vi "8_Find roots of the quadratic equation.vi"() -> ()   [LabVIEW 2018]
panel:
  out "SUBTRACT":dbl
  out "ADD":dbl
  in  "C":dbl
  in  "B":dbl
  in  "A":dbl
  # "WAP to find roots of the quadratic equation"
  # "Ax^2 + Bx + C= 0"
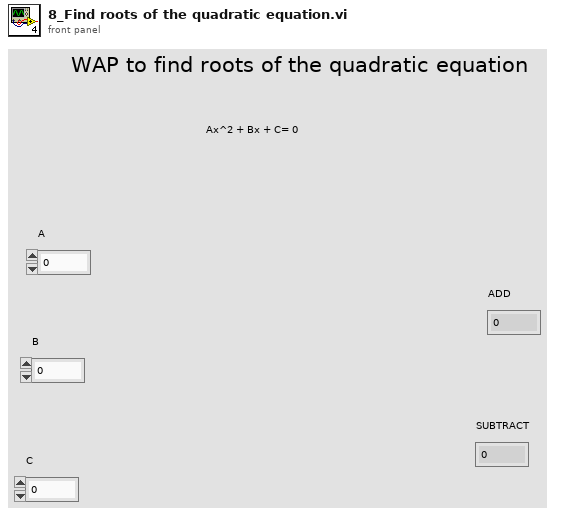
[diagram p1: front panel]
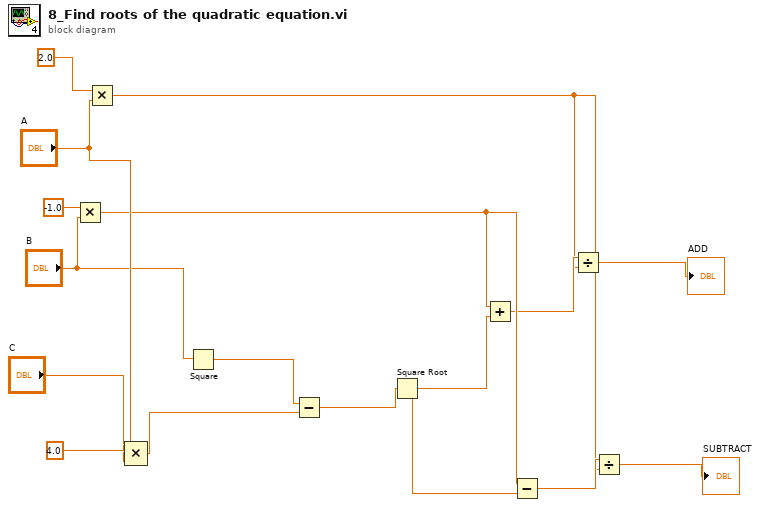
[diagram p0: block diagram]
diagram:
  n1 = Multiply(x=-1.0, y="B") -> (x*y=w6:dbl)
  n2 = Multiply(x=2.0, y="A") -> (x*y=w3:dbl)
  n3 = Compound Arithmetic op=MULTIPLY(4.0 ("result"), "A", "C") -> (w13:dbl)
  n4 = Square(x="B") -> (x^2=w14:dbl)
  n5 = Subtract(x=w14, y=w13) -> (x-y=w12:dbl)
  n6 = Square Root(x=w12) -> (sqrt(x)=w11:dbl)
  n7 = Add(x=w6, y=w11) -> (x+y=w5:dbl)
  n8 = Subtract(x=w6, y=w11) -> (x-y=w4:dbl)
  n9 = Divide(x=w5, y=w3) -> (x/y=→"ADD":dbl)
  n10 = Divide(x=w4, y=w3) -> (x/y=→"SUBTRACT":dbl)
